vi "TxRollback_Core.vi"(8 "error in (no error)":errorcluster, 11 "DbConnection in":refnum<class "ORM_DBC_dotNet.lvclass">) -> (0 "error out":errorcluster, 3 "DbConnection out":refnum<class "ORM_DBC_dotNet.lvclass">)   [LabVIEW 2020, in "ORM_DBC_dotNet.lvlib" / "ORM_DBC_dotNet.lvclass"]
uses:
  ORM_DBC_dotNet.lvclass
  ORM_DBC_dotNet.lvclass/ORM_DBC_dotNet.ctl
  Read transactions.vi
  Write transactions.vi
  System.Data
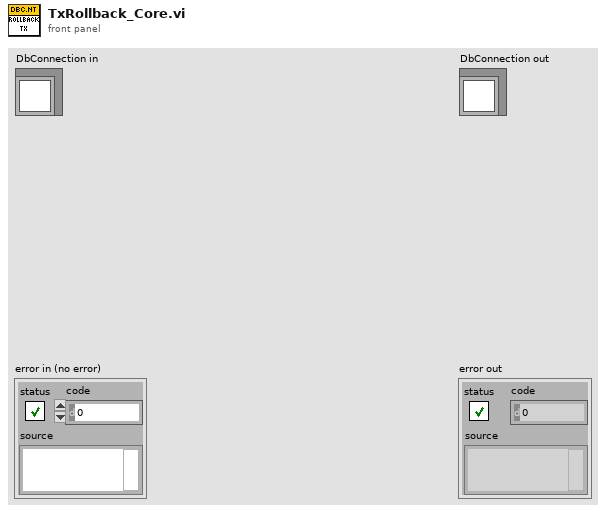
[diagram p1: front panel]
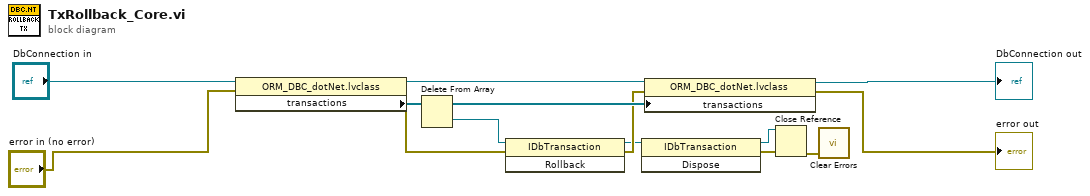
[diagram p0: block diagram]
diagram:
  n1 = property class="ORM_DBC_dotNet.lvclass"(reference="DbConnection in", error in="error in (no error)") -> (reference out=w8:refnum<class "ORM_DBC_dotNet.lvclass">, error out=w6:errorcluster, "transactions"=w10:refnum<k24>[])
  n2 = Delete From Array(array=w10) -> (deleted portion=w9:refnum<k24>, array with subset deleted=w7:refnum<k24>[])  [unwired: 2 in]
  n3 = invoke class="IDbTransaction" method="Rollback"(reference=w9, error in=w6) -> (reference out=w4:refnum<k24>, error out=w5:errorcluster)  [unwired: 1 in, 1 out]
  n4 = invoke class="IDbTransaction" method="Dispose"(reference=w4) -> (reference out=w2:refnum<k24>, error out=w3:errorcluster)  [unwired: 2 in, 1 out]
  n5 = property class="ORM_DBC_dotNet.lvclass"(reference=w8, error in=w5, "transactions"=w7) -> (reference out=→"DbConnection out":refnum<class "ORM_DBC_dotNet.lvclass">, error out=→"error out":errorcluster)
  n6 = Close Reference(reference=w2, error in (no error)=w3) -> (error out=w1:errorcluster)
  n7 = call <vilib>:"Clear Errors.vi"("error in (no error)"=w1) -> ()  [unwired: 5 in, 2 out]
